vi "EPOS2N~3.VI"() -> ()   [LabVIEW 2017]
doc: "Example of controlling 1 EPOS2 drive in current mode."
uses:
  <vilib>/addons/Maxon Motor/EPOS2 CANopen/EPOS2 Support Files/Typedefs/EPOS2 Data Output Current.ctl
  <vilib>/addons/Maxon Motor/EPOS2 CANopen/EPOS2 Support Files/Typedefs/EPOS2 Status Word PVM.ctl
  <vilib>/addons/Maxon Motor/EPOS2 CANopen/CANopen/sbCANopenBaseClass.lvclass
  <vilib>/addons/Maxon Motor/EPOS2 CANopen/EPOS2 Support Files/Typedefs/EPOS2 Control Word PVM.ctl
  <vilib>/Platform/TimedLoop/XDataNode/timing_clust.ctl
  <vilib>/Platform/TimedLoop/XDataNode/nitl_modes.ctl
  <vilib>/Platform/TimedLoop/XDataNode/wakeup.ctl
  <vilib>/addons/Maxon Motor/EPOS2 CANopen/EPOS2 Support Files/Polymorphic SubVIs/Write PDO/EPOS2 Current Mode Write.vi
  <vilib>/addons/Maxon Motor/EPOS2 CANopen/EPOS2 Support Files/Polymorphic SubVIs/Read PDO/EPOS2 Current Mode Read.vi
  <vilib>/Platform/TimedLoop/XDataNode/XDataNode.xnode
  <vilib>/Platform/TimedLoop/XDataNode/XDNodeRunTimeDep.lvlib
  <vilib>/addons/Maxon Motor/EPOS2 CANopen/EPOS2 Library.lvlib
panel:
  in  "Current 2":i32(slide) scale=-1000.0..1000.0
  out "Node ID 4":u8
  in  "index 2":i32
  out "for 1":i32
  in  "length":i32=4
  in  "index":i32
  out "motors":refnum<class "sbCANopenBaseClass.lvclass">[](array[class])
  out "Finished Late? [i-1]":bool
  out "element":refnum<class "sbCANopenBaseClass.lvclass">
  out "Status 2":T1
  out "Data Output 2":T2
  out "Node ID 3":u8
  in  "Current":i32(slide) scale=-1000.0..1000.0
  in  "stop":bool
  # "This Example VI demonstrates how to control the current of an EPOS2 drive using a CANopen interface.\n\nThis VI must be run from a LabVIEW Project. An Example Projects can be found at: \nC:\\Program Files\\National Instruments\\LabVIEW 2015\\examples\\Maxon Motor\\Maxon EPOS2\nor simliar relative path to current LabVIEW version install location for all opperating systems"
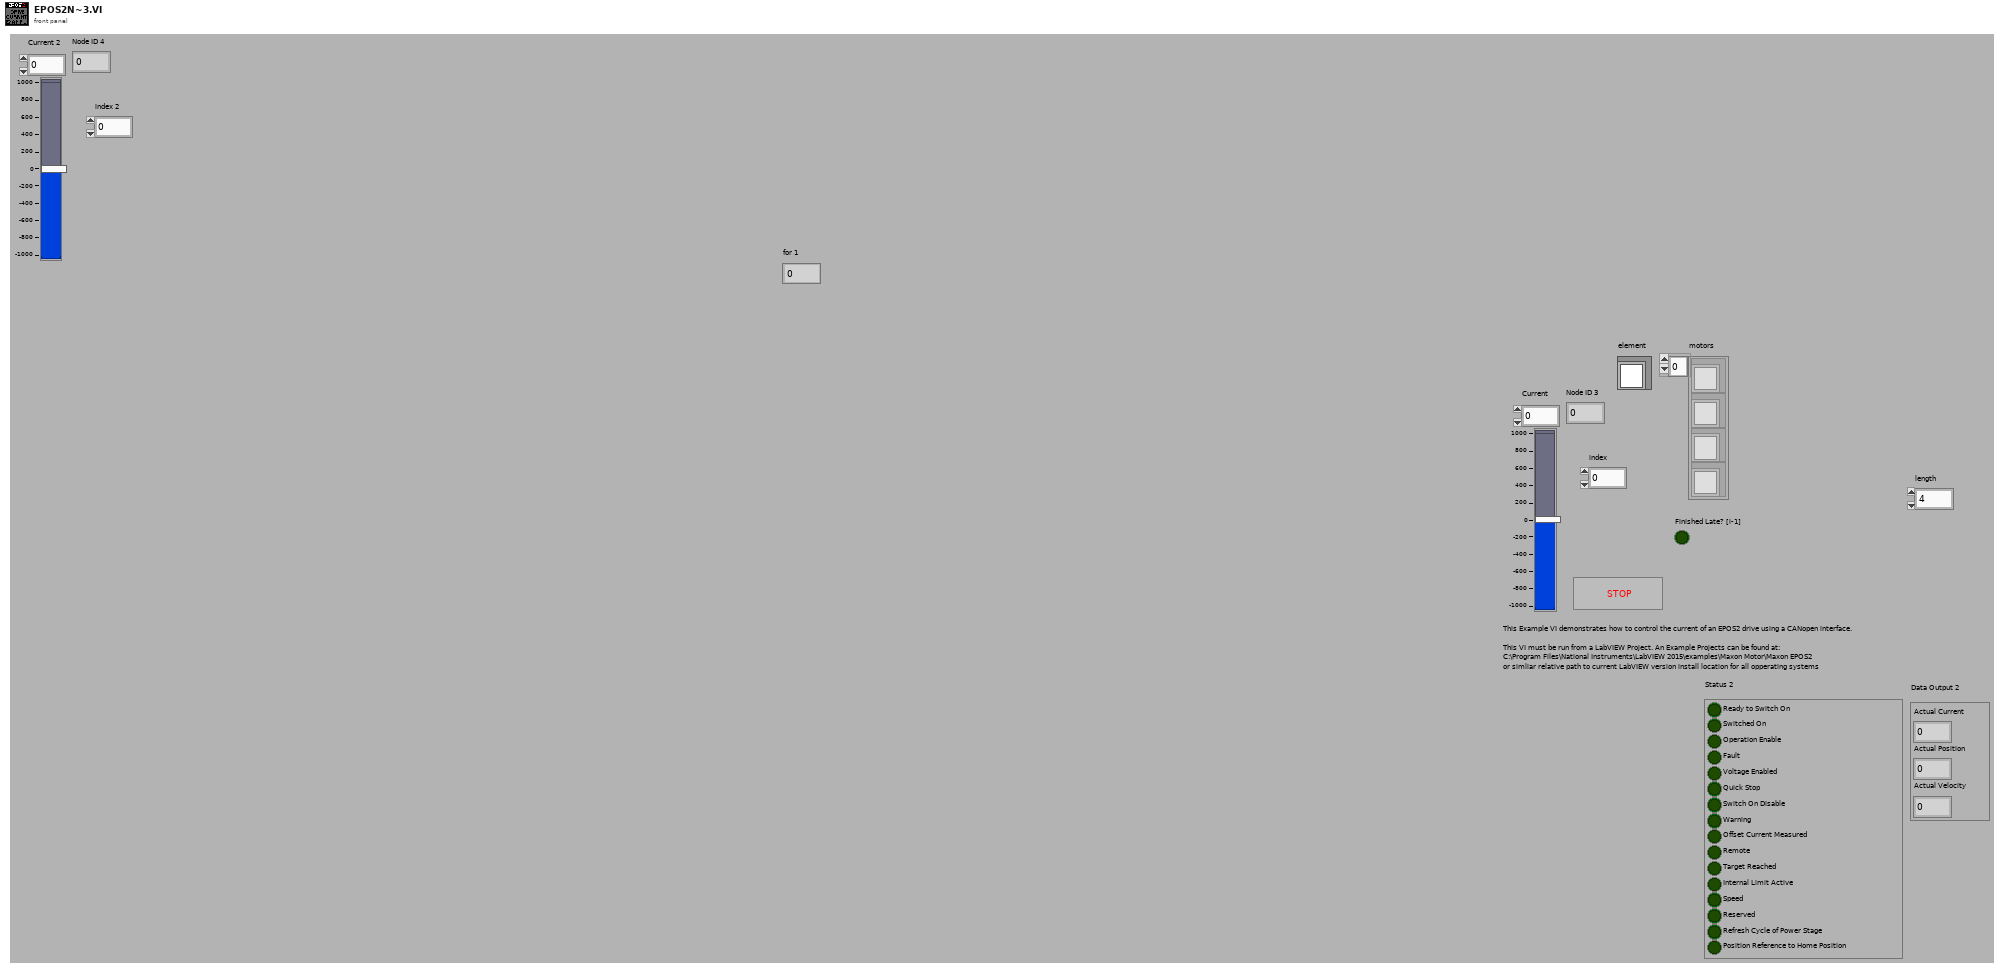
[diagram p1: front panel]
types:
  T1 = typedef "EPOS2 Library.lvlib/EPOS2 Status Word PVM.ctl" = cluster{"Ready to Switch On":bool, "Switched On":bool, "Operation Enable":bool, "Fault":bool, "Voltage Enabled":bool, "Quick Stop":bool, "Switch On Disable":bool, "Warning":bool, "Offset Current Measured":bool, "Remote":bool, "Target Reached":bool, "Internal Limit Active":bool, "Speed":bool, "Reserved":bool, "Refresh Cycle of Power Stage":bool, "Position Reference to Home Position":bool}
  T2 = typedef "EPOS2 Library.lvlib/EPOS2 Data Output Current.ctl" = cluster{"Actual Current":i16, "Actual Position":i32, "Actual Velocity":i32}
  T3 = typedef "EPOS2 Library.lvlib/EPOS2 Control Word PVM.ctl" = cluster{"Switch On":bool, "Enable Voltage":bool, "Quick Stop":bool, "Enable Operation":bool, "Reserved 0":bool, "Reserved 1":bool, "Reserved 2":bool, "Fault Reset":bool, "Halt":bool}
  T4 = typedef "XDNodeRunTimeDep.lvlib/timing_clust.ctl" = cluster{"Expected End [f-1]":u64, "Actual End [f-1]":u64, "Finished Late? [f-1]":bool, "Expected End [i-1]":u64, "Actual End [i-1]":u64, "Finished Late? [i-1]":bool, "Expected Start [i]":u64, "Actual Start [i]":u64, "Expected Start [f]":u64, "Actual Start [f]":u64, "Source Name":string, "Structure Name":string, "Period":i64, "Deadline":i64, "Offset":i64, "Start":i64, "Priority":i32, "Timeout":i32, "Mode":T5, "Wakeup Reason":T6, "Error":errorcluster, "Source Type":string, "Secondary Source Type":string, "Global End Time":u64, "Global Start Time":u64, "Frame Duration":u64, "Iteration Duration":u64, "Assigned CPU":i32, "I/O Scan Engine Mode":u32}
  T5 = typedef "XDNodeRunTimeDep.lvlib/nitl_modes.ctl" = enum32{"No Change", "Process missed periods, maintain original phase", "Discard missed periods, maintain original phase", "Process missed periods, ignore original phase", "Discard missed periods, ignore original phase"}
  T6 = typedef "XDNodeRunTimeDep.lvlib/wakeup.ctl" = enum32{"Normal", "Aborted", "Asynchronous wakeup", "Timing source error", "Timed loop error", "Timeout"}
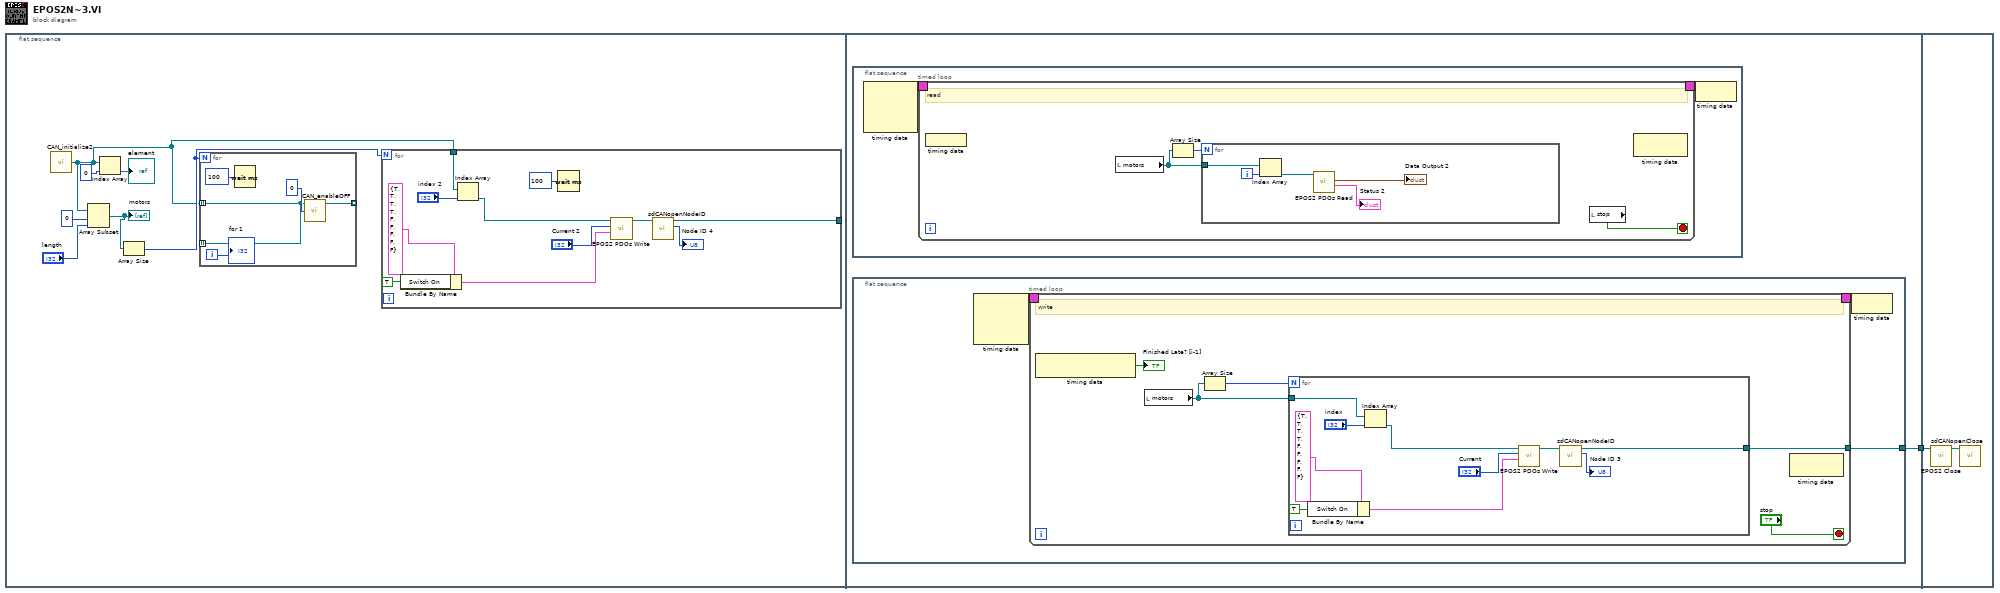
[diagram p0: block diagram]
diagram:
  n1 = flat-sequence {
    tunnel: [w25] -> w1
    tunnel: w1 -> [w63]
    frame #0 {
      n2 = call "CAN_initialize2.vi"() -> ("Array"=w2:refnum<class "sbCANopenBaseClass.lvclass">[])  [unwired: 3 in, 2 out]
      n3 = Array Subset(array=w2, index=0 ("length"), length="length") -> (w4:refnum<class "sbCANopenBaseClass.lvclass">[])
      "motors" <- w4
      n4 = Index Array(array=w2, index=0) -> (element=→"element":refnum<class "sbCANopenBaseClass.lvclass">)
      n5 = Array Size(array=w4) -> (size(s)=w3:i32)
      n6 = for {
        N: w3 -> [_]
        tunnel: [w23] -> _ mode=indexing
        tunnel: w2 -> [w23] mode=indexing
        tunnel: [w20] -> _ mode=indexing
        i -> [w21]
        n7 = Wait (ms)(milliseconds to wait=u32 100) -> ()  [unwired: 1 out]
        n8 = call "CAN_enableOFF.vi"("Current"=0, "sbCANopenBaseClass in"=w23) -> ("CANopen Session Out"=w20:refnum<class "sbCANopenBaseClass.lvclass">)  [unwired: 2 in, 1 out]
        "for 1" <- w21
      }
      n9 = for {
        N: w3 -> [_]
        tunnel: [w16] -> _
        tunnel: w2 -> [w10]
        n10 = Bundle By Name(cluster=T3 {"Switch On"=TRUE, "Enable Voltage"=TRUE, "Quick Stop"=TRUE, "Enable Operation"=TRUE, "Reserved 0"=FALSE, "Reserved 1"=FALSE, "Reserved 2"=FALSE, "Fault Reset"=FALSE, "Halt"=FALSE} ("Control Word"), "Switch On"=TRUE) -> (w13:T3)
        n11 = Index Array(array=w10, index="index 2") -> (element=w12:refnum<class "sbCANopenBaseClass.lvclass">)
        n12 = Wait (ms)(milliseconds to wait=u32 100) -> ()  [unwired: 1 out]
        n13 = call-poly <vilib>:"EPOS2 PDOs Write.vi"("Control Word"=w13, "Current"="Current 2", "CANopen Session In"=w12) -> ("CANopen Session Out"=w17:refnum<class "sbCANopenBaseClass.lvclass">)  [unwired: 7 in, 1 out]
        n14 = call-dynamic "sdCANopenNodeID.vi"("sbCANopenBaseClass in"=w17) -> ("Node ID"=→"Node ID 4":u8, "sbCANopenBaseClass out"=w16:refnum<class "sbCANopenBaseClass.lvclass">)  [unwired: 9 in]
      }
    }
    frame #1 {
      n15 = flat-sequence {
        frame #0 {
          n16 = node-c288() -> (w50:T4)  [unwired: 1 in, 2 out]
          n17 = timed-loop {
            timing: w50 -> [_]
            timing-out: [_] -> w49
            stop <- w53 stop-if-true
            # "read"
            n18 = node-c288() -> ()  [unwired: 1 out]
            n19 = local read "motors"() -> (w51:refnum<class "sbCANopenBaseClass.lvclass">[])
            n20 = Array Size(array=w51) -> (size(s)=w52:i32)
            n21 = for {
              N: w52 -> [_]
              tunnel: w51 -> [w55]
              i -> [w54]
              n22 = Index Array(array=w55, index=w54) -> (element=w56:refnum<class "sbCANopenBaseClass.lvclass">)
              n23 = call-poly <vilib>:"EPOS2 PDOs Read.vi"("CANopen Session In"=w56) -> ("Statusword"=→"Status 2":T1, "Data Output"=→"Data Output 2":T2)  [unwired: 7 in, 2 out]
            }
            n24 = local read "stop"() -> (w53:bool)
            n25 = node-c288() -> ()  [unwired: 2 out]
          }
          n26 = node-c288(w49) -> ()
        }
      }
      n27 = flat-sequence {
        tunnel: [w26] -> w25
        frame #0 {
          n28 = node-c288() -> (w28:T4)  [unwired: 2 in, 1 out]
          n29 = timed-loop {
            timing: w28 -> [_]
            timing-out: [_] -> w27
            tunnel: [w32] -> w26
            stop <- "stop" stop-if-true
            # "write"
            n30 = node-c288() -> (→"Finished Late? [i-1]":bool)  [unwired: 1 out]
            n31 = local read "motors"() -> (w29:refnum<class "sbCANopenBaseClass.lvclass">[])
            n32 = Array Size(array=w29) -> (size(s)=w30:i32)
            n33 = for {
              N: w30 -> [_]
              tunnel: [w40] -> w32
              tunnel: w29 -> [w39]
              n34 = Bundle By Name(cluster=T3 {"Switch On"=TRUE, "Enable Voltage"=TRUE, "Quick Stop"=TRUE, "Enable Operation"=TRUE, "Reserved 0"=FALSE, "Reserved 1"=FALSE, "Reserved 2"=FALSE, "Fault Reset"=FALSE, "Halt"=FALSE} ("Control Word"), "Switch On"=TRUE) -> (w36:T3)
              n35 = Index Array(array=w39, index="index") -> (element=w35:refnum<class "sbCANopenBaseClass.lvclass">)
              n36 = call-poly <vilib>:"EPOS2 PDOs Write.vi"("Control Word"=w36, "Current"="Current", "CANopen Session In"=w35) -> ("CANopen Session Out"=w41:refnum<class "sbCANopenBaseClass.lvclass">)  [unwired: 7 in, 1 out]
              n37 = call-dynamic "sdCANopenNodeID.vi"("sbCANopenBaseClass in"=w41) -> ("Node ID"=→"Node ID 3":u8, "sbCANopenBaseClass out"=w40:refnum<class "sbCANopenBaseClass.lvclass">)  [unwired: 9 in]
            }
            n38 = node-c288() -> ()  [unwired: 2 out]
          }
          n39 = node-c288(w27) -> ()
        }
      }
    }
    frame #2 {
      n40 = call <vilib>:"EPOS2 Close.vi"("CANopen Session In"=w63) -> ("CANopen Session Out"=w64:refnum<class "sbCANopenBaseClass.lvclass">)  [unwired: 3 in, 7 out]
      n41 = call-dynamic "sdCANopenClose.vi"("sbCANopenBaseClass in"=w64) -> ()  [unwired: 9 in, 2 out]
    }
  }
